vi "Tutorial - Tags and Properties.vi"   [LabVIEW 2020]
doc: "Use this VI to teach you how to use Tags and Properties with the Nominal IO LabVIEW Client."
uses:
  e58265c6-ef23-4a71-adf2-d0c15f719ea7.vi
  b9193784-df40-4e33-a64f-e62c0c03439d.vi
  8f762aeb-0866-454b-9e21-5f24372cd99a.vi
  21bdf8d0-e820-4d0b-9592-2a1ddc50d7ec.vi
  753263d8-b5d8-460c-ad4f-d510297832fd.vi
  4024a2c0-490d-4e64-9d09-648060e46672.vi
  Nominal Client/Nominal Client.lvclass
panel:
  # "Take a look on the block diagram\nCtrl + E"
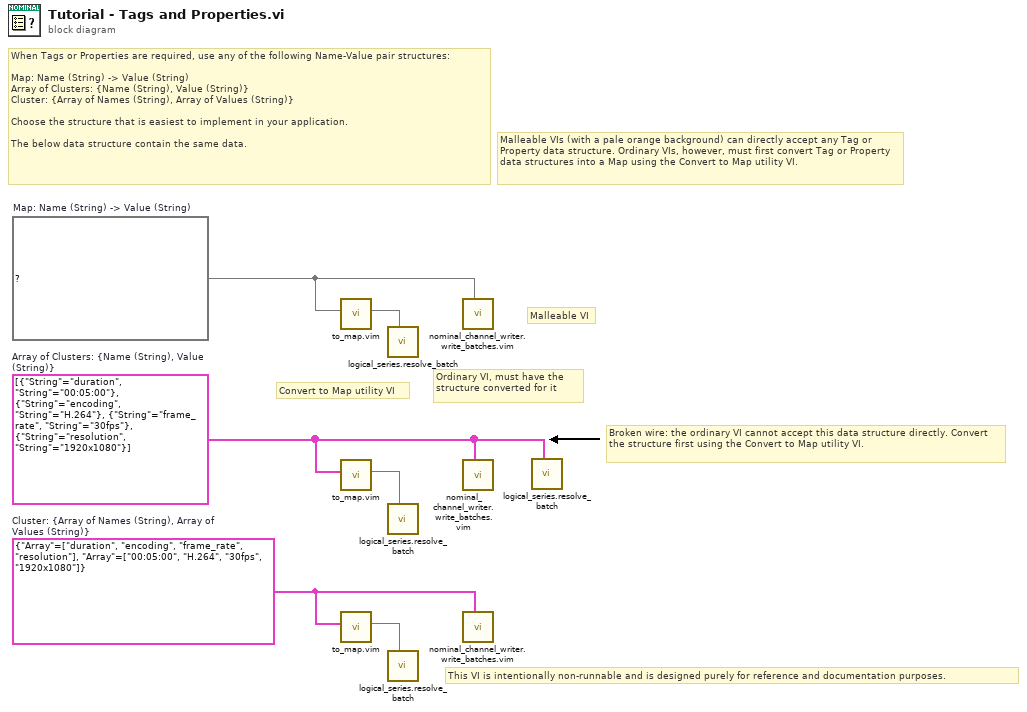
[diagram p0: block diagram]
diagram:
  w5 = cluster{"Array":string[], "Array":string[]} {"Array"=["duration", "encoding", "frame_rate", "resolution"], "Array"=["00:05:00", "H.264", "30fps", "1920x1080"]}  # Cluster: {Array of Names (String), Array of Values (String)}
  w1 = cluster{"String":string, "String":string}[] [{"String"="duration", "String"="00:05:00"}, {"String"="encoding", "String"="H.264"}, {"String"="frame_rate", "String"="30fps"}, {"String"="resolution", "String"="1920x1080"}]  # Array of Clusters: {Name (String), Value (String)}
  w6 = map{string, string} {"duration"="00:05:00", "encoding"="H.264", "frame_rate"="30fps", "resolution"="1920x1080"}  # Map: Name (String) -> Value (String)
  # "This VI is intentionally non-runnable and is designed purely for reference and documentation purposes."
  # "Broken wire: the ordinary VI cannot accept this data structure directly. Convert the structure first using the Convert to Map utility VI."
  # "Convert to Map utility VI"
  # "Ordinary VI, must have the structure converted for it"
  # "Malleable VI"
  # "Malleable VIs (with a pale orange background) can directly accept any Tag or Property data structure. Ordinary VIs, however, must first convert Tag or Property data structures into a Map using the Convert to Map utility VI."
  # "When Tags or Properties are required, use any of the following Name-Value pair structures:\n\nMap: Name (String) -> Value (String)\nArray of Clusters: {Name (String), Value (String)}\nCluster: {Array of Names (String), Array of Values (String)}\n\nChoose the structure that is easiest to implement in your application.\n\nThe below data structure contain the same data."
  n1 = call "to_map.vim"("Map"=w6) -> ("Map out"=w4:map{string, string})  [unwired: 10 in]
  n2 = call "to_map.vim"("Map"=w1) -> ("Map out"=w3:map{string, string})  [unwired: 10 in]
  n3 = call "to_map.vim"("Map"=w5) -> ("Map out"=w2:map{string, string})  [unwired: 10 in]
  n4 = call "logical_series.resolve_batch.vi"("tags"=w4) -> ()  [unwired: 8 in, 3 out]
  n5 = call "logical_series.resolve_batch.vi"("tags"=w3) -> ()  [unwired: 8 in, 3 out]
  n6 = call "logical_series.resolve_batch.vi"("tags"=w2) -> ()  [unwired: 8 in, 3 out]
  n7 = call "nominal_channel_writer.write_batches.vim"("Tags"=w6) -> ()  [unwired: 8 in, 3 out]
  n8 = call "nominal_channel_writer.write_batches.vim"("Tags"=w1) -> ()  [unwired: 8 in, 3 out]
  n9 = call "nominal_channel_writer.write_batches.vim"("Tags"=w5) -> ()  [unwired: 8 in, 3 out]
  n10 = call "logical_series.resolve_batch.vi"("tags"=w1) -> ()  [unwired: 8 in, 3 out]
